vi "Reset SRQ.vi"(8 "error in (no error)":errorcluster, 10 "Address (0)":i32, 11 "VISA resource name":refnum<visa-resource-name>) -> (0 "error out":errorcluster, 3 "VISA resource name out":refnum<visa-resource-name>)   [LabVIEW 2016, in "Environment Chamber.lvlib" / "Climatic Chamber.lvlib"]
doc: "<b>SRQ status setting</B>\n\nClears the SRQ (Service Request) status."
uses:
  Climatic Chamber.lvlib
panel:
  out "NACK":bool
  out "Error":bool
  out "ACK":bool
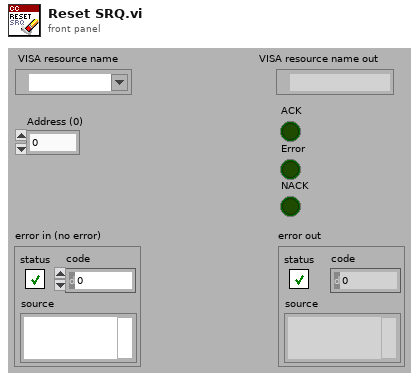
[diagram p1: front panel]
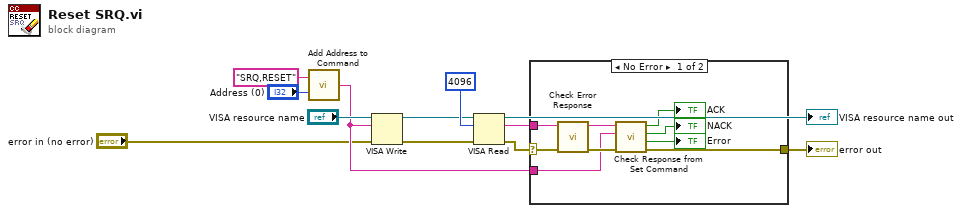
[diagram p0: block diagram]
diagram:
  n1 = call "Add Address to Command.vi"("Address (0)"="Address (0)", "Command"="SRQ,RESET") -> ("Command OUT"=w3:string)
  n2 = VISA Write(VISA resource name="VISA resource name", write buffer=w3, error in (no error)="error in (no error)") -> (VISA resource name out=w10:refnum<visa-resource-name>, error out=w9:errorcluster)  [unwired: 1 out]
  n3 = VISA Read(VISA resource name=w10, byte count=u32 4096, error in (no error)=w9) -> (VISA resource name out=→"VISA resource name out":refnum<visa-resource-name>, read buffer=w5:string, error out=w6:errorcluster)  [unwired: 1 out]
  n4 = case shown="No Error" w6 {
    selector: w6 -> [w20 w22]
    tunnel: w5 -> [w21 _]
    tunnel: [w16 w22] -> w4
    tunnel: w3 -> [w17 _]
    frame No Error {
      n5 = call "Check Error Response.vi"("error in (no error)"=w20, "read String"=w21) -> ("error out"=w19:errorcluster, "String out"=w18:string)  [unwired: 7 in, 1 out]
      n6 = call "Check Response from Set Command.vi"("error in (no error)"=w19, "Command"=w17, "Response"=w18) -> ("error out"=w16:errorcluster, "Error"=→"Error":bool, "NACK"=→"NACK":bool, "ACK"=→"ACK":bool)  [unwired: 5 in]
    }
    frame Error {
    }
  }
  "error out" <- w4
